vi "ReadWiringsNode.vi"(8 "Error In":errorcluster, 11 "Keithley2602 Node In":refnum<k20>) -> (0 "Error Out":errorcluster, 2 "Wirings":T1[](array[typedef]), 3 "Keithley2602 Node Out":refnum<k20>)   [LabVIEW 2013]
uses:
  driver/Public/Controls/SMUSense.ctl
  <vilib>/xml/NI_XML.lvlib
  driver/Keithley-2602.lvlib
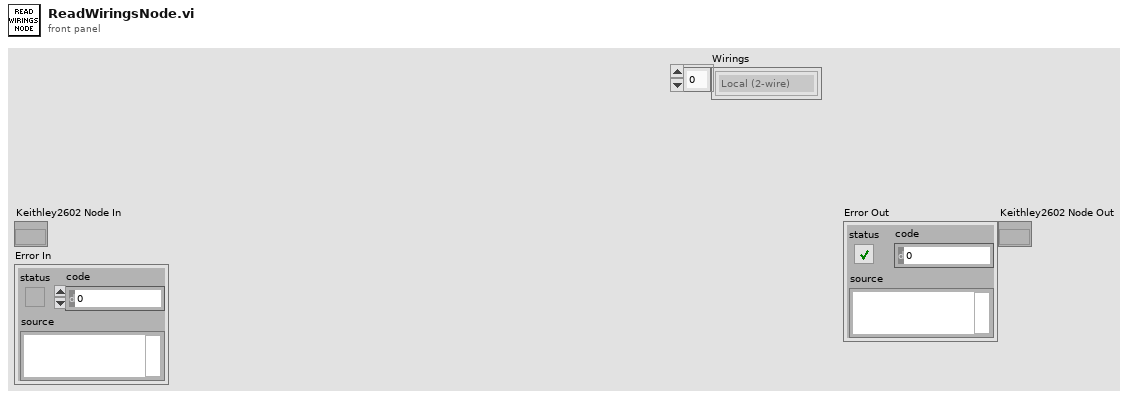
[diagram p1: front panel]
types:
  T1 = typedef "Keithley-2602.lvlib/SMUSense.ctl" = enum16{"Local (2-wire)", "Remote (4-wire)", "Calibration"}
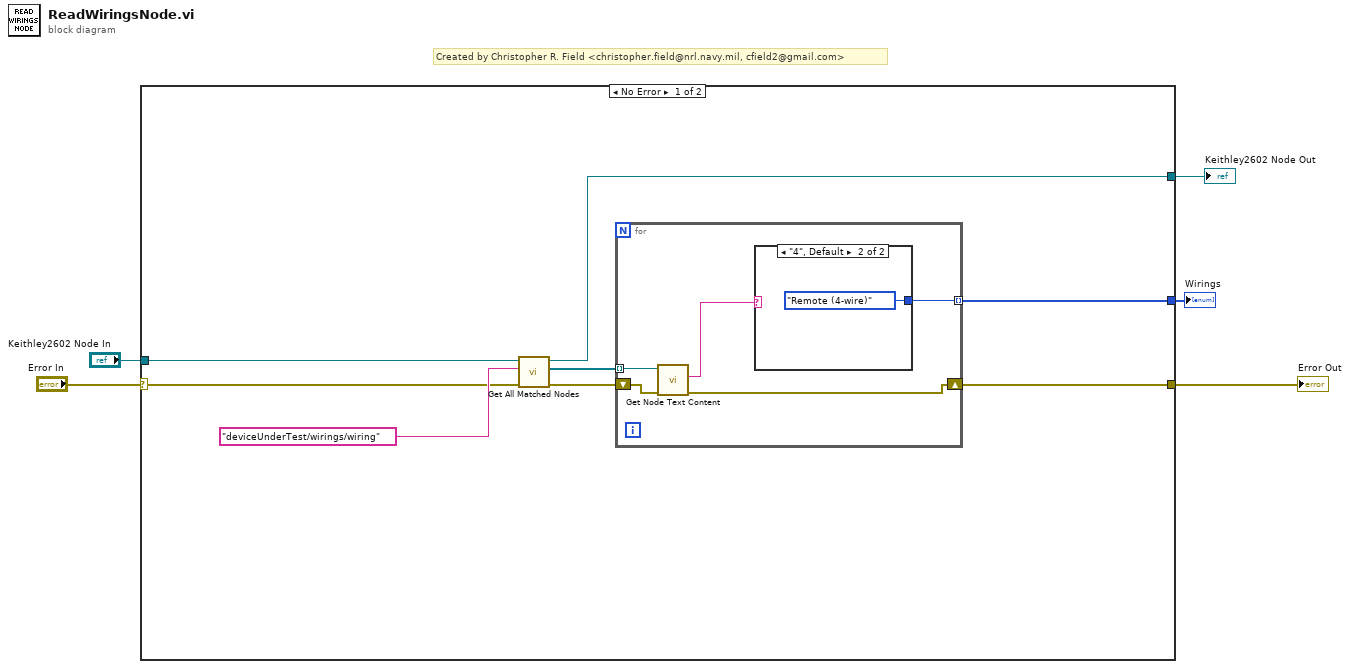
[diagram p0: block diagram]
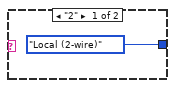
[diagram p2: hidden frame]
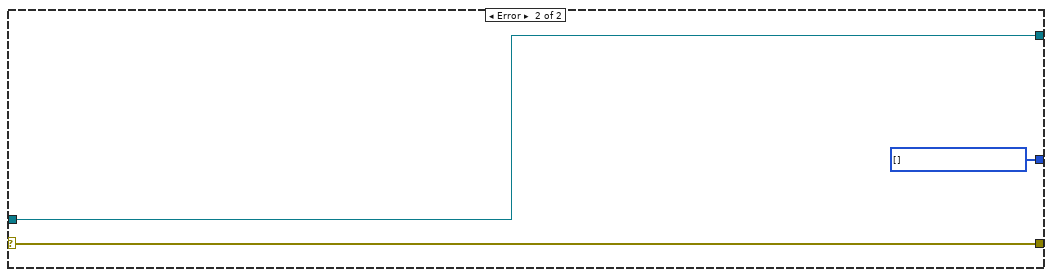
[diagram p3: hidden frame]
diagram:
  # "Created by Christopher R. Field <christopher.field@nrl.navy.mil, cfield2@gmail.com>"
  n1 = case shown="No Error" "Error In" {
    selector: "Error In" -> [w7 w22]
    tunnel: "Keithley2602 Node In" -> [w10 w23]
    tunnel: [w9 w22] -> w4
    tunnel: [w8 w23] -> w3
    tunnel: [w6 w21] -> w1
    frame No Error {
      n2 = call <vilib>:"Get All Matched Nodes.vi"("error in (no error)"=w7, "XPath expression"="deviceUnderTest/wirings/wiring", "node in"=w10) -> ("error out"=w11:errorcluster, "node result array"=w12:refnum<k20>[], "node out"=w8:refnum<k20>)  [unwired: 6 in]
      n3 = for {
        tunnel: w12 -> [w18] mode=indexing
        shift-right: [w16] -> w9
        shift-left: w11 -> [w17]
        tunnel: [w14] -> w6 mode=indexing
        n4 = call <vilib>:"Get Node Text Content.vi"("error in (no error)"=w17, "node in"=w18) -> ("error out"=w16:errorcluster, "node text"=w15:string)  [unwired: 7 in, 1 out]
        n5 = case shown="\"4\", Default" w15 {
          tunnel: [SMUSense."Local (2-wire)" ("SMU Sense") SMUSense."Remote (4-wire)" ("SMU Sense")] -> w14
          frame "2" {
          }
          frame "4", Default {
          }
        }
      }
    }
    frame Error {
      w21 = T1[] [] items=["Local (2-wire)", "Remote (4-wire)", "Calibration"]
    }
  }
  "Error Out" <- w4
  "Keithley2602 Node Out" <- w3
  "Wirings" <- w1
